vi "WhatHindbraintoMidbrainFilterCalibrate.vi"(3 "WhatAroundMe?":cluster{"T":dbl, "Range":dbl, "Bearing":dbl}[](array[cluster])) -> (1 "WhatAroundMe? Clean":cluster{"T":dbl, "Range":dbl, "Bearing":dbl}[](array[cluster]))   [LabVIEW 2010]
doc: "This subVI takes raw I16 \"What is around me?\" data from the hindbrain and filters and calibrates it to become clean double data for the Midbrain. Cluster is:\n\nt=time\nr=range\nb=bearing"
uses:
  <vilib>/Analysis/3filter.llb/Filter Passband Type.ctl
  <vilib>/Analysis/3filter.llb/Butterworth Filter (DBL).vi
  <vilib>/Analysis/NI_AALBase.lvlib
panel:
  out "Waveform Graph":dbl[][](graph)
  # "This subVI filters and \nand calabrates the\nWhat is arounf me? data \nfrom the hindbrain"
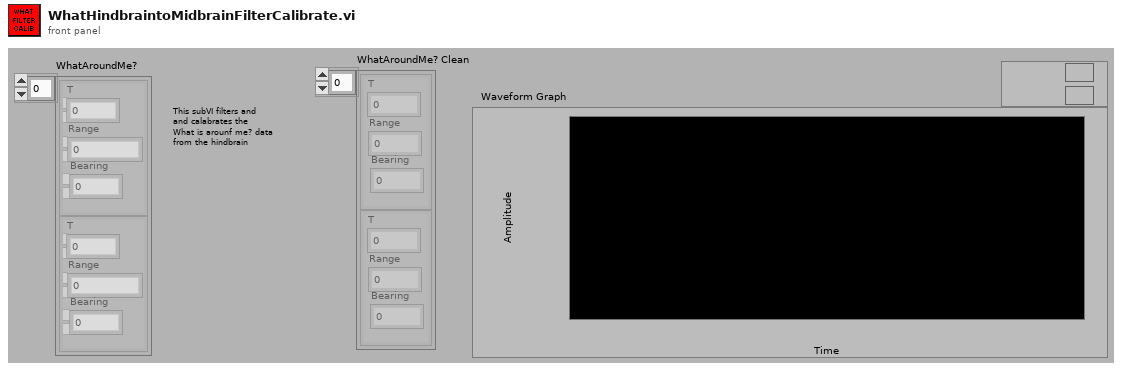
[diagram p1: front panel]
types:
  T1 = typedef "NI_AALBase.lvlib/Filter Passband Type.ctl" = enum32{"Lowpass", "Highpass", "Bandpass", "Bandstop"}
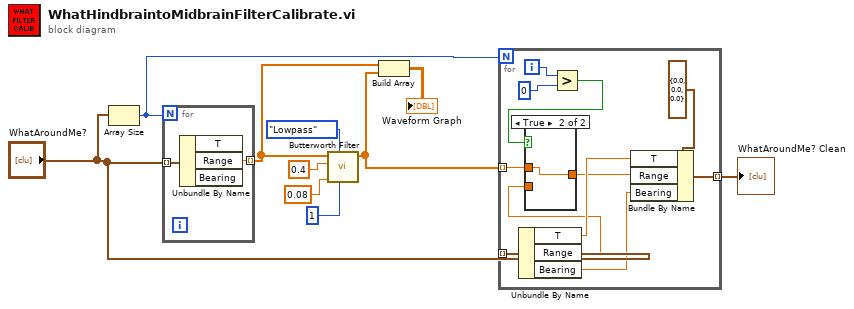
[diagram p0: block diagram]
diagram:
  n1 = Array Size(array="WhatAroundMe?") -> (size(s)=w3:i32)
  n2 = for {
    N: w3 -> [_]
    tunnel: [w12] -> _ mode=indexing
    tunnel: "WhatAroundMe?" -> [w12] mode=indexing
    tunnel: [w11] -> w9 mode=indexing
    n3 = Unbundle By Name(w12) -> ("Range"=w11:dbl)  [unwired: 2 out]
  }
  n4 = call-poly <vilib>:"Butterworth Filter.vi"("order"=1, "filter type"=Filter_Passband_Type."Lowpass", "low cutoff freq: fl"=0.08, "sampling freq: fs"=0.4, "X"=w9) -> ("Filtered X"=w4:dbl[])  [unwired: 3 in, 1 out]
  n5 = Build Array(w9, w4) -> (→"Waveform Graph":dbl[][])
  n6 = for {
    N: w3 -> [_]
    tunnel: w4 -> [w14] mode=indexing
    tunnel: "WhatAroundMe?" -> [w21] mode=indexing
    tunnel: [w22] -> w2 mode=indexing
    i -> [w18]
    n7 = Unbundle By Name(w21) -> ("T"=w20:dbl, "Range"=w15:dbl, "Bearing"=w19:dbl)
    n8 = Greater?(x=w18, y=0) -> (0:w16:bool)
    n9 = case shown="True" w16 {
      tunnel: w15 -> [w24 _]
      tunnel: w14 -> [_ w25]
      tunnel: [w24 w25] -> w13
      frame False {
      }
      frame True {
      }
    }
    n10 = Bundle By Name(cluster=cluster{"T":dbl, "Range":dbl, "Bearing":dbl} {"T"=0.0, "Range"=0.0, "Bearing"=0.0} ("Cluster"), "T"=w20, "Range"=w13, "Bearing"=w19) -> (w22:cluster{"T":dbl, "Range":dbl, "Bearing":dbl})
  }
  "WhatAroundMe? Clean" <- w2
